vi "main functie.vi"(11 "input array   4":dbl[](array[numeric])) -> (2 "Array":i32[](array[numeric]), 3 "Numeric":i32)   [LabVIEW 2019]
uses:
  <vilib>/myRIO/Common/Instrument Driver Framework/Utilities/typedefs/Analog Scaling Constants.ctl
  <vilib>/myRIO/Common/Instrument Driver Framework/Utilities/typedefs/Analog Scaling Constants List.ctl
  <vilib>/myRIO/Common/Instrument Driver Framework/myRIO v1.0/AO/typedefs/AO Channels Enum.ctl
  <vilib>/myRIO/Common/Instrument Driver Framework/myRIO v1.0/AO/typedefs/AO Channels List.ctl
  <vilib>/myRIO/Common/Instrument Driver Framework/Utilities/typedefs/Generic FPGA Reference.ctl
  <vilib>/myRIO/Common/Instrument Driver Framework/Utilities/typedefs/myRIO v1.0 Reference.ctl
  <vilib>/myRIO/Common/Instrument Driver Framework/Utilities/typedefs/Hardware Version Enum.ctl
  <vilib>/myRIO/Common/Instrument Driver Framework/Utilities/typedefs/myRIO Generic Hardware Reference.ctl
  <vilib>/myRIO/Instrument Drivers/Onboard IO/AO/typedefs/AO Reference.ctl
  <vilib>/myRIO/Instrument Drivers/Onboard IO/AO/AO.lvlib
  <vilib>/myRIO/Instrument Drivers/Onboard IO/AO/vis/Write.vi
  <vilib>/userDefined/High Color/nirio_resource_hc.ctl
  <vilib>/myRIO/Common/Instrument Driver Framework/myRIO v1.0/AO/vis/myRIO v1.1 Open AO.vi
  <vilib>/myRIO/Instrument Drivers/Onboard IO/AO/vis/myRIO AO Open.xnode
  <vilib>/myRIO/Common/Instrument Driver Framework/Utilities/vis/Is FPGA Ref Available.vi
  <vilib>/myRIO/Express VI/Onboard IO/AO/AO Express VI.xnode
panel:
  in  "Numeric 4":dbl
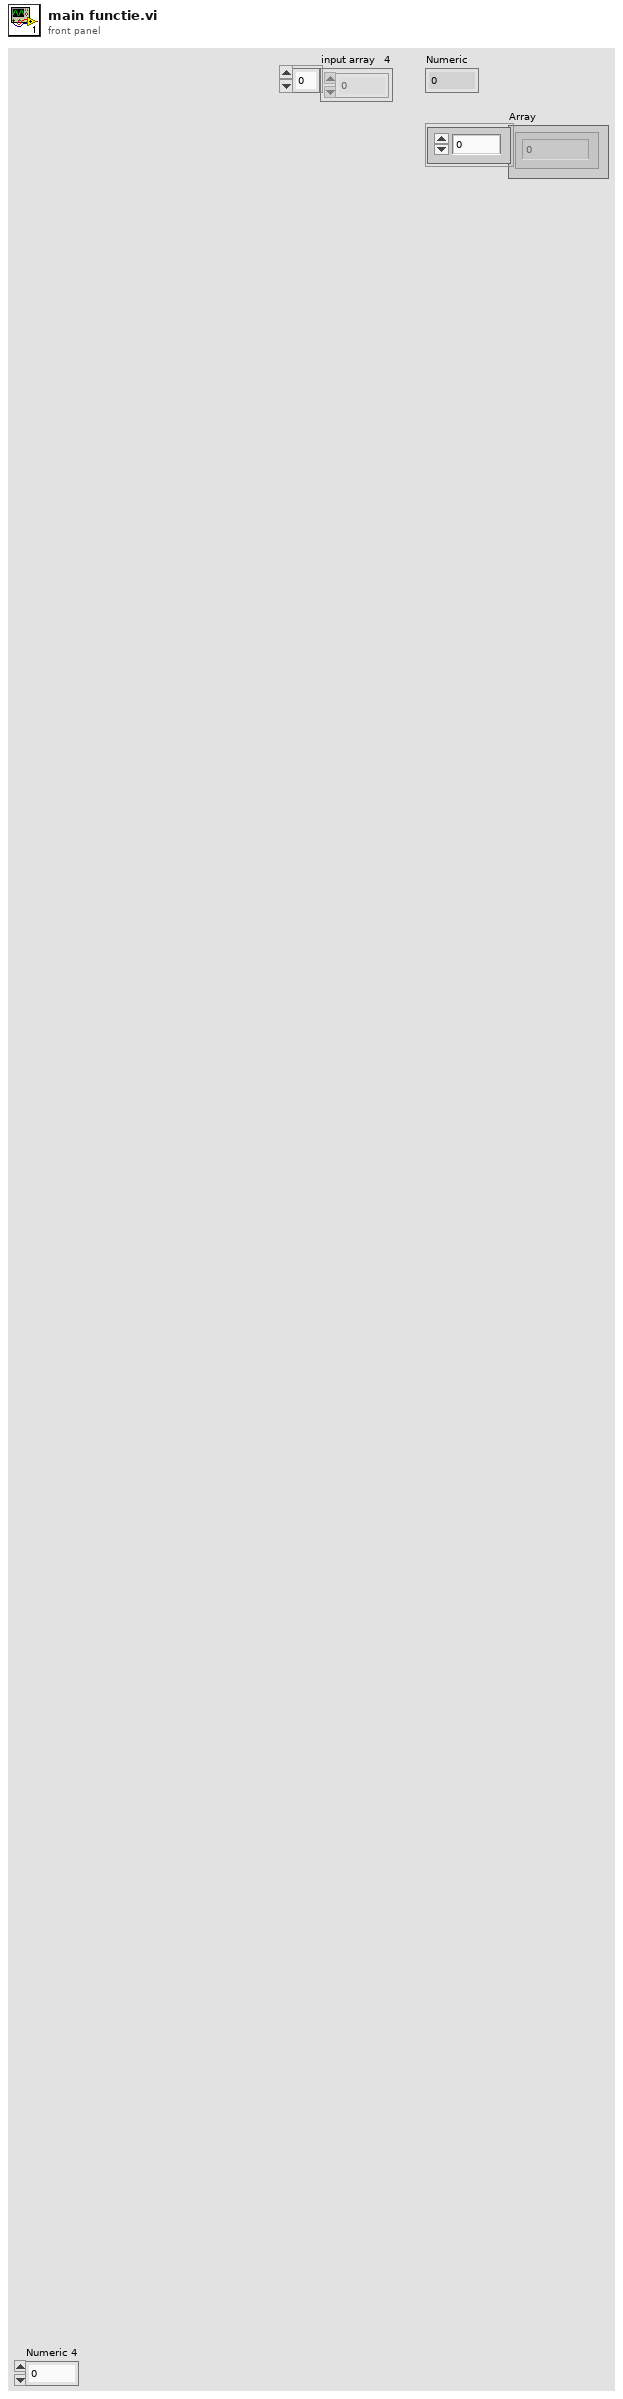
[diagram p1: front panel]
types:
  T1 = typedef "AO.lvlib/AO Reference.ctl" = cluster{"myRIO Reference":T2, "AO Channel List":T6, "AO Scaling Constant List":T8}
  T2 = typedef "myRIO Generic Hardware Reference.ctl" = cluster{"myRIO Model":T3, "myRIO Hardware Reference":T4}
  T3 = typedef "Hardware Version Enum.ctl" = enum16{"Unknown", "myRIO-1900", "myRIO-1950", "roboRIO", "NI ELVIS RIO CM", "ELVIS III"}
  T4 = typedef "myRIO v1.0 Reference.ctl" = cluster{"Generic FPGA Reference":T5, "Allow multiple opens":bool}
  T5 = typedef "Generic FPGA Reference.ctl" = refnum<k20>
  T6 = typedef "AO Channels List.ctl" = T7[]
  T7 = typedef "AO Channels Enum.ctl" = enum16{"Not Connected", "AudioOut/Left", "AudioOut/Right", "C/AO0", "C/AO1", "A/AO0", "A/AO1", "B/AO0", "B/AO1"}
  T8 = typedef "Analog Scaling Constants List.ctl" = T9[]
  T9 = typedef "Analog Scaling Constants.ctl" = cluster{"LSB Weight (Volts)":dbl, "Offset (Volts)":dbl, "Signed?":bool}
  T10 = typedef "nirio_resource_hc.ctl" = tag
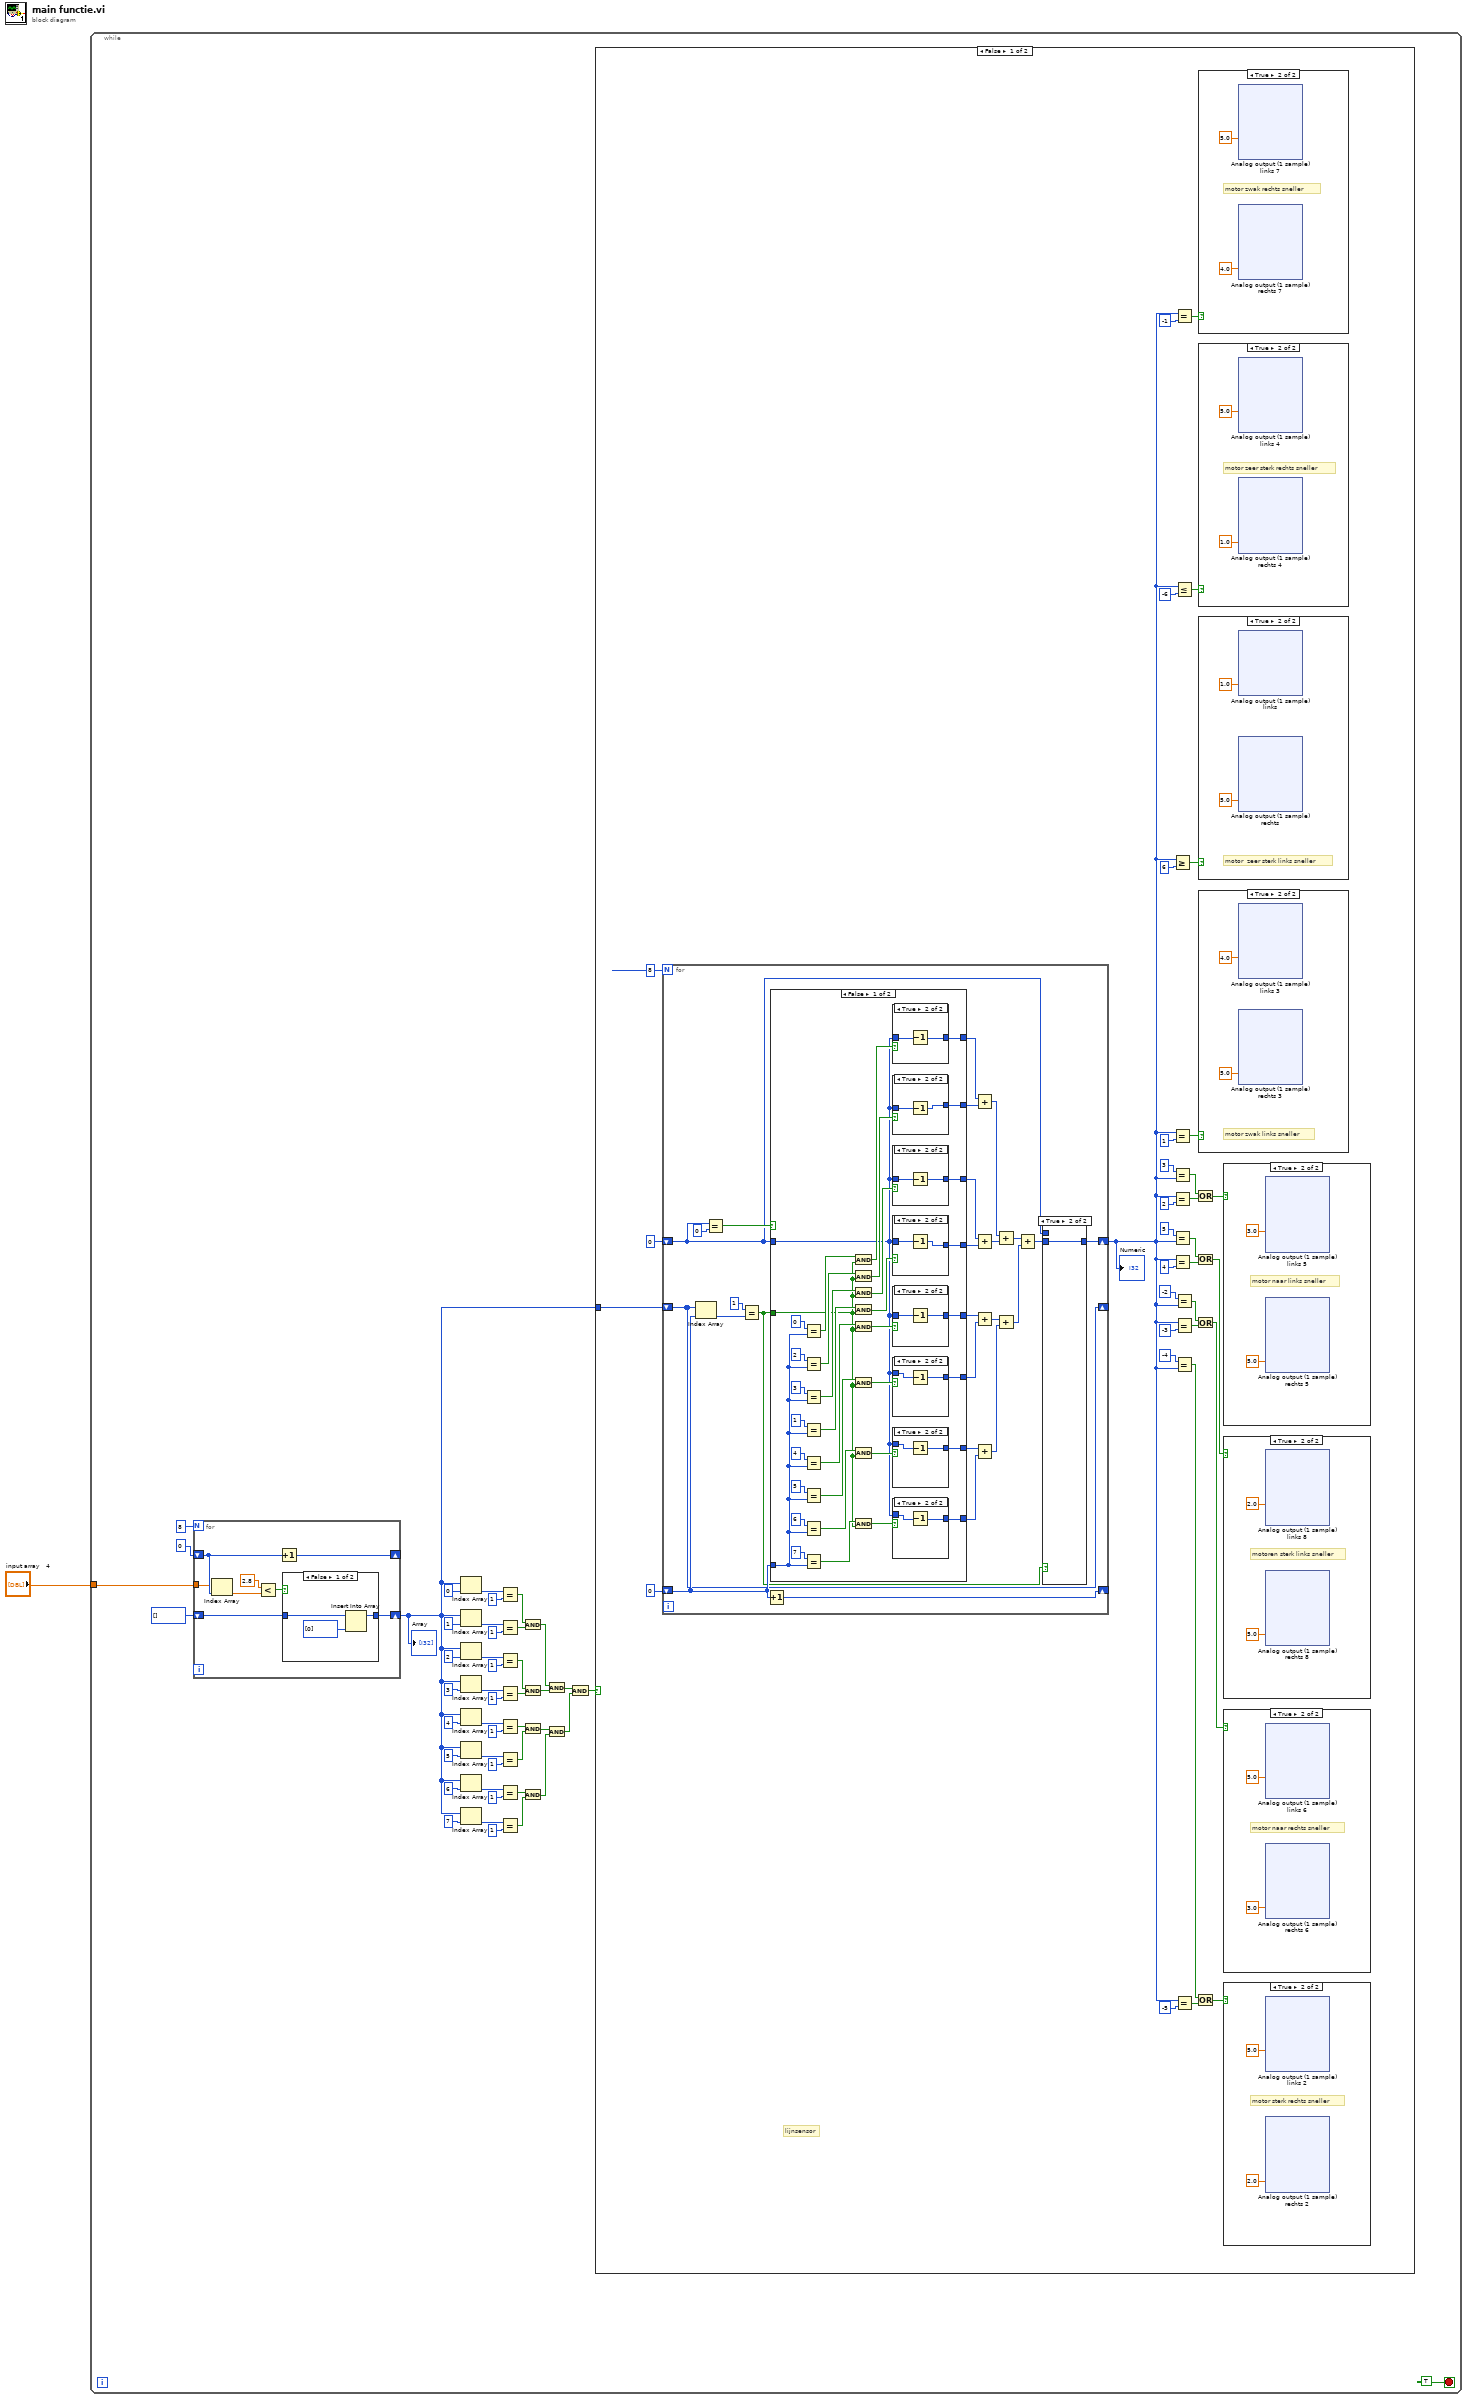
[diagram p0: block diagram]
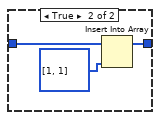
[diagram p2: hidden frame]
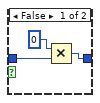
[diagram p12: hidden frame]
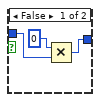
[diagram p13: hidden frame]
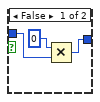
[diagram p14: hidden frame]
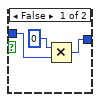
[diagram p15: hidden frame]
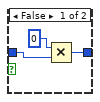
[diagram p16: hidden frame]
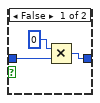
[diagram p17: hidden frame]
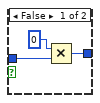
[diagram p18: hidden frame]
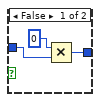
[diagram p19: hidden frame]
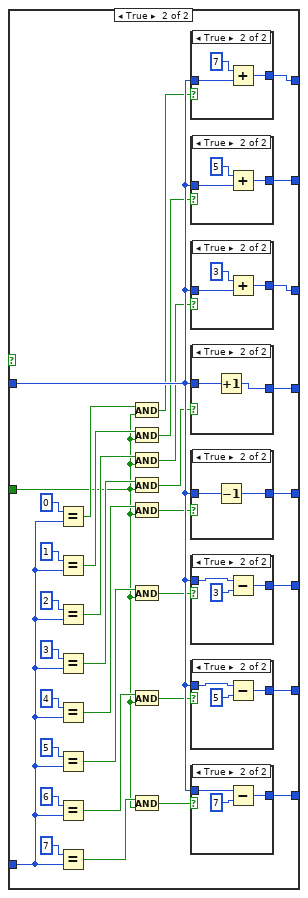
[diagram p20: hidden frame]
diagram:
  n1 = while {
    tunnel: "input array   4" -> [w46]
    stop <- TRUE stop-if-true
    n2 = for {
      N: 8 -> [_]
      shift-right: [w53] -> w45
      shift-left: i32[] [] -> [w54]
      shift-right: [w50] -> _
      shift-left: 0 -> [w49]
      tunnel: w46 -> [w47]
      n3 = Index Array(array=w47, index=w49) -> (element=w48:dbl)
      n4 = Less?(x=2.8, y=w48) -> (x < y?=w52:bool)
      n5 = Increment(x=w49) -> (x+1=w50:i32)
      n6 = case shown="False" w52 {
        tunnel: w54 -> [w56 w58]
        tunnel: [w57 w60] -> w53
        frame False {
          n7 = Insert Into Array(array=w56, new element=i32[] [0]) -> (w57:i32[])  [unwired: 1 in]
        }
        frame True {
          n8 = Insert Into Array(array=w58, new element=i32[] [1, 1]) -> (w60:i32[])  [unwired: 1 in]
        }
      }
    }
    "Array" <- w45
    n9 = Index Array(array=w45, index=0) -> (element=w24:i32)
    n10 = Index Array(array=w45, index=1) -> (element=w3:i32)
    n11 = Index Array(array=w45, index=2) -> (element=w9:i32)
    n12 = Index Array(array=w45, index=3) -> (element=w6:i32)
    n13 = Index Array(array=w45, index=4) -> (element=w12:i32)
    n14 = Index Array(array=w45, index=5) -> (element=w15:i32)
    n15 = Index Array(array=w45, index=6) -> (element=w18:i32)
    n16 = Index Array(array=w45, index=7) -> (element=w21:i32)
    n17 = Equal?(x=w24, y=1) -> (x = y?=w27:bool)
    n18 = Equal?(x=w3, y=1) -> (x = y?=w28:bool)
    n19 = Equal?(x=w9, y=1) -> (x = y?=w29:bool)
    n20 = Equal?(x=w6, y=1) -> (x = y?=w30:bool)
    n21 = Equal?(x=w12, y=1) -> (x = y?=w31:bool)
    n22 = Equal?(x=w15, y=1) -> (x = y?=w32:bool)
    n23 = Equal?(x=w18, y=1) -> (x = y?=w33:bool)
    n24 = Equal?(x=w21, y=1) -> (x = y?=w34:bool)
    n25 = And(x=w27, y=w28) -> (x .and. y?=w35:bool)
    n26 = And(x=w29, y=w30) -> (x .and. y?=w36:bool)
    n27 = And(x=w31, y=w32) -> (x .and. y?=w37:bool)
    n28 = And(x=w33, y=w34) -> (x .and. y?=w38:bool)
    n29 = And(x=w35, y=w36) -> (x .and. y?=w39:bool)
    n30 = And(x=w37, y=w38) -> (x .and. y?=w40:bool)
    n31 = And(x=w39, y=w40) -> (x .and. y?=w41:bool)
    n32 = case shown="False" w41 {
      tunnel: w45 -> [w62 _]
      frame False {
        # "lijnsensor"
        n33 = for {
          N: 8 -> [_]
          shift-right: [w712] -> _
          shift-left: 0 -> [w726]
          shift-right: [w704] -> w61
          shift-left: 0 -> [w705]
          shift-right: [w717] -> _
          shift-left: w62 -> [w717]
          n34 = Index Array(array=w717, index=w726) -> (element=w716:i32)
          n35 = Equal?(x=w705, y=0) -> (x = y?=w713:bool)
          n36 = Equal?(x=1, y=w716) -> (x = y?=w703:bool)
          n37 = Increment(x=w726) -> (x+1=w712:i32)
          n38 = case shown="False" w713 {
            tunnel: w726 -> [w736 w822]
            tunnel: [w730 w821] -> w725
            tunnel: [w737 w820] -> w724
            tunnel: [w738 w819] -> w723
            tunnel: [w739 w818] -> w722
            tunnel: w705 -> [w729 w817]
            tunnel: w703 -> [w735 w808]
            tunnel: [w733 w807] -> w711
            tunnel: [w734 w806] -> w710
            tunnel: [w731 w805] -> w708
            tunnel: [w732 w804] -> w707
            frame False {
              n39 = Equal?(x=0, y=w736) -> (x = y?=w756:bool)
              n40 = Equal?(x=2, y=w736) -> (x = y?=w762:bool)
              n41 = Equal?(x=3, y=w736) -> (x = y?=w763:bool)
              n42 = Equal?(x=1, y=w736) -> (x = y?=w748:bool)
              n43 = Equal?(x=4, y=w736) -> (x = y?=w760:bool)
              n44 = Equal?(x=5, y=w736) -> (x = y?=w761:bool)
              n45 = Equal?(x=6, y=w736) -> (x = y?=w759:bool)
              n46 = Equal?(x=7, y=w736) -> (x = y?=w758:bool)
              n47 = And(x=w756, y=w735) -> (x .and. y?=w740:bool)
              n48 = And(x=w762, y=w735) -> (x .and. y?=w742:bool)
              n49 = And(x=w763, y=w735) -> (x .and. y?=w743:bool)
              n50 = And(x=w748, y=w735) -> (x .and. y?=w741:bool)
              n51 = And(x=w760, y=w735) -> (x .and. y?=w744:bool)
              n52 = And(x=w761, y=w735) -> (x .and. y?=w745:bool)
              n53 = And(x=w759, y=w735) -> (x .and. y?=w746:bool)
              n54 = And(x=w758, y=w735) -> (x .and. y?=w747:bool)
              n55 = case shown="True" w740 {
                tunnel: [w765 w768] -> w734
                tunnel: w729 -> [w764 w767]
                frame False {
                  n56 = Multiply(x=0, y=w764) -> (x*y=w765:i32)
                }
                frame True {
                  n57 = Decrement(x=w767) -> (x-1=w768:i32)
                }
              }
              n58 = case shown="True" w742 {
                tunnel: [w796 w797] -> w733
                tunnel: w729 -> [w795 w798]
                frame False {
                  n59 = Multiply(x=0, y=w795) -> (x*y=w796:i32)
                }
                frame True {
                  n60 = Decrement(x=w798) -> (x-1=w797:i32)
                }
              }
              n61 = case shown="True" w743 {
                tunnel: [w790 w793] -> w732
                tunnel: w729 -> [w789 w792]
                frame False {
                  n62 = Multiply(x=0, y=w789) -> (x*y=w790:i32)
                }
                frame True {
                  n63 = Decrement(x=w792) -> (x-1=w793:i32)
                }
              }
              n64 = case shown="True" w741 {
                tunnel: [w800 w803] -> w731
                tunnel: w729 -> [w799 w802]
                frame False {
                  n65 = Multiply(x=0, y=w799) -> (x*y=w800:i32)
                }
                frame True {
                  n66 = Decrement(x=w802) -> (x-1=w803:i32)
                }
              }
              n67 = case shown="True" w744 {
                tunnel: [w785 w788] -> w730
                tunnel: w729 -> [w784 w787]
                frame False {
                  n68 = Multiply(x=0, y=w784) -> (x*y=w785:i32)
                }
                frame True {
                  n69 = Decrement(x=w787) -> (x-1=w788:i32)
                }
              }
              n70 = case shown="True" w745 {
                tunnel: [w775 w778] -> w737
                tunnel: w729 -> [w774 w777]
                frame False {
                  n71 = Multiply(x=0, y=w774) -> (x*y=w775:i32)
                }
                frame True {
                  n72 = Decrement(x=w777) -> (x-1=w778:i32)
                }
              }
              n73 = case shown="True" w746 {
                tunnel: [w780 w783] -> w738
                tunnel: w729 -> [w779 w782]
                frame False {
                  n74 = Multiply(x=0, y=w779) -> (x*y=w780:i32)
                }
                frame True {
                  n75 = Decrement(x=w782) -> (x-1=w783:i32)
                }
              }
              n76 = case shown="True" w747 {
                tunnel: [w769 w773] -> w739
                tunnel: w729 -> [w770 w772]
                frame False {
                  n77 = Multiply(x=0, y=w770) -> (x*y=w769:i32)
                }
                frame True {
                  n78 = Decrement(x=w772) -> (x-1=w773:i32)
                }
              }
            }
            frame True {
              n79 = Equal?(x=0, y=w822) -> (x = y?=w831:bool)
              n80 = Equal?(x=1, y=w822) -> (x = y?=w823:bool)
              n81 = Equal?(x=2, y=w822) -> (x = y?=w837:bool)
              n82 = Equal?(x=3, y=w822) -> (x = y?=w838:bool)
              n83 = Equal?(x=4, y=w822) -> (x = y?=w835:bool)
              n84 = Equal?(x=5, y=w822) -> (x = y?=w836:bool)
              n85 = Equal?(x=6, y=w822) -> (x = y?=w834:bool)
              n86 = Equal?(x=7, y=w822) -> (x = y?=w833:bool)
              n87 = And(x=w831, y=w808) -> (x .and. y?=w809:bool)
              n88 = And(x=w823, y=w808) -> (x .and. y?=w810:bool)
              n89 = And(x=w837, y=w808) -> (x .and. y?=w811:bool)
              n90 = And(x=w838, y=w808) -> (x .and. y?=w812:bool)
              n91 = And(x=w835, y=w808) -> (x .and. y?=w813:bool)
              n92 = And(x=w836, y=w808) -> (x .and. y?=w814:bool)
              n93 = And(x=w834, y=w808) -> (x .and. y?=w815:bool)
              n94 = And(x=w833, y=w808) -> (x .and. y?=w816:bool)
              n95 = case shown="True" w809 {
                tunnel: w817 -> [w839 w843]
                tunnel: [w840 w842] -> w806
                frame False {
                  n96 = Multiply(x=0, y=w839) -> (x*y=w840:i32)
                }
                frame True {
                  n97 = Add(x=7, y=w843) -> (x+y=w842:i32)
                }
              }
              n98 = case shown="True" w810 {
                tunnel: w817 -> [w879 w882]
                tunnel: [w880 w883] -> w807
                frame False {
                  n99 = Multiply(x=0, y=w879) -> (x*y=w880:i32)
                }
                frame True {
                  n100 = Add(x=5, y=w882) -> (x+y=w883:i32)
                }
              }
              n101 = case shown="True" w811 {
                tunnel: w817 -> [w873 w877]
                tunnel: [w874 w876] -> w804
                frame False {
                  n102 = Multiply(x=0, y=w873) -> (x*y=w874:i32)
                }
                frame True {
                  n103 = Add(x=3, y=w877) -> (x+y=w876:i32)
                }
              }
              n104 = case shown="True" w812 {
                tunnel: w817 -> [w869 w872]
                tunnel: [w868 w871] -> w805
                frame False {
                  n105 = Multiply(x=0, y=w869) -> (x*y=w868:i32)
                }
                frame True {
                  n106 = Increment(x=w872) -> (x+1=w871:i32)
                }
              }
              n107 = case shown="True" w813 {
                tunnel: w817 -> [w863 w867]
                tunnel: [w864 w866] -> w821
                frame False {
                  n108 = Multiply(x=0, y=w863) -> (x*y=w864:i32)
                }
                frame True {
                  n109 = Decrement(x=w867) -> (x-1=w866:i32)
                }
              }
              n110 = case shown="True" w814 {
                tunnel: w817 -> [w852 w854]
                tunnel: [w851 w856] -> w820
                frame False {
                  n111 = Multiply(x=0, y=w852) -> (x*y=w851:i32)
                }
                frame True {
                  n112 = Subtract(x=w854, y=3) -> (x-y=w856:i32)
                }
              }
              n113 = case shown="True" w815 {
                tunnel: w817 -> [w858 w860]
                tunnel: [w857 w861] -> w819
                frame False {
                  n114 = Multiply(x=0, y=w858) -> (x*y=w857:i32)
                }
                frame True {
                  n115 = Subtract(x=w860, y=5) -> (x-y=w861:i32)
                }
              }
              n116 = case shown="True" w816 {
                tunnel: w817 -> [w845 w848]
                tunnel: [w846 w849] -> w818
                frame False {
                  n117 = Multiply(x=0, y=w845) -> (x*y=w846:i32)
                }
                frame True {
                  n118 = Subtract(x=w848, y=7) -> (x-y=w849:i32)
                }
              }
            }
          }
          n119 = Add(x=w710, y=w711) -> (x+y=w709:i32)
          n120 = Add(x=w707, y=w708) -> (x+y=w706:i32)
          n121 = Add(x=w725, y=w724) -> (x+y=w720:i32)
          n122 = Add(x=w723, y=w722) -> (x+y=w721:i32)
          n123 = Add(x=w709, y=w706) -> (x+y=w719:i32)
          n124 = Add(x=w720, y=w721) -> (x+y=w718:i32)
          n125 = Add(x=w719, y=w718) -> (x+y=w702:i32)
          n126 = case shown="True" w703 {
            tunnel: w705 -> [w727 _]
            tunnel: [w727 w728] -> w704
            tunnel: w702 -> [_ w728]
            frame False {
            }
            frame True {
            }
          }
        }
        "Numeric" <- w61
        n127 = Greater Or Equal?(x=w61, y=6) -> (x >= y?=w88:bool)
        n128 = Equal?(x=w61, y=1) -> (x = y?=w89:bool)
        n129 = Equal?(x=3, y=w61) -> (x = y?=w79:bool)
        n130 = Equal?(x=w61, y=2) -> (x = y?=w80:bool)
        n131 = Equal?(x=5, y=w61) -> (x = y?=w83:bool)
        n132 = Equal?(x=w61, y=4) -> (x = y?=w84:bool)
        n133 = Equal?(x=w61, y=-1) -> (x = y?=w67:bool)
        n134 = Less Or Equal?(x=w61, y=-6) -> (x <= y?=w65:bool)
        n135 = Equal?(x=-2, y=w61) -> (x = y?=w73:bool)
        n136 = Equal?(x=w61, y=-3) -> (x = y?=w74:bool)
        n137 = Equal?(x=-4, y=w61) -> (x = y?=w69:bool)
        n138 = Equal?(x=w61, y=-5) -> (x = y?=w70:bool)
        n139 = Or(x=w79, y=w80) -> (x .or. y?=w77:bool)
        n140 = Or(x=w83, y=w84) -> (x .or. y?=w85:bool)
        n141 = Or(x=w73, y=w74) -> (x .or. y?=w66:bool)
        n142 = Or(x=w69, y=w70) -> (x .or. y?=w63:bool)
        n143 = case shown="True" w67 {
          frame False {
          }
          frame True {
            # "motor zwak rechts sneller"
            n144 = xnode "Analog output (1 sample) links 7"("A/AO0 (Pin 2)"=5.0) -> ()  [unwired: 1 in, 1 out]
            n145 = xnode "Analog output (1 sample) rechts 7"("A/AO0 (Pin 2)"=4.0) -> ()  [unwired: 1 in, 1 out]
          }
        }
        n146 = case shown="True" w65 {
          frame False {
          }
          frame True {
            # "motor zeer sterk rechts sneller"
            n147 = xnode "Analog output (1 sample) links 4"("A/AO0 (Pin 2)"=5.0) -> ()  [unwired: 1 in, 1 out]
            n148 = xnode "Analog output (1 sample) rechts 4"("A/AO0 (Pin 2)"=1.0) -> ()  [unwired: 1 in, 1 out]
          }
        }
        n149 = case shown="True" w88 {
          frame False {
          }
          frame True {
            # "motor  zeer sterk links sneller"
            n150 = xnode "Analog output (1 sample) links"("A/AO0 (Pin 2)"=1.0) -> ()  [unwired: 1 in, 1 out]
            n151 = xnode "Analog output (1 sample) rechts"("A/AO0 (Pin 2)"=5.0) -> ()  [unwired: 1 in, 1 out]
          }
        }
        n152 = case shown="True" w89 {
          frame False {
          }
          frame True {
            # "motor zwak links sneller"
            n153 = xnode "Analog output (1 sample) links 3"("A/AO0 (Pin 2)"=4.0) -> ()  [unwired: 1 in, 1 out]
            n154 = xnode "Analog output (1 sample) rechts 3"("A/AO0 (Pin 2)"=5.0) -> ()  [unwired: 1 in, 1 out]
          }
        }
        n155 = case shown="True" w77 {
          frame False {
          }
          frame True {
            # "motor naar links sneller"
            n156 = xnode "Analog output (1 sample) links 5"("A/AO0 (Pin 2)"=3.0) -> ()  [unwired: 1 in, 1 out]
            n157 = xnode "Analog output (1 sample) rechts 5"("A/AO0 (Pin 2)"=5.0) -> ()  [unwired: 1 in, 1 out]
          }
        }
        n158 = case shown="True" w85 {
          frame False {
          }
          frame True {
            # "motoren sterk links sneller"
            n159 = xnode "Analog output (1 sample) links 8"("A/AO0 (Pin 2)"=2.0) -> ()  [unwired: 1 in, 1 out]
            n160 = xnode "Analog output (1 sample) rechts 8"("A/AO0 (Pin 2)"=5.0) -> ()  [unwired: 1 in, 1 out]
          }
        }
        n161 = case shown="True" w66 {
          frame False {
          }
          frame True {
            # "motor naar rechts sneller"
            n162 = xnode "Analog output (1 sample) links 6"("A/AO0 (Pin 2)"=5.0) -> ()  [unwired: 1 in, 1 out]
            n163 = xnode "Analog output (1 sample) rechts 6"("A/AO0 (Pin 2)"=3.0) -> ()  [unwired: 1 in, 1 out]
          }
        }
        n164 = case shown="True" w63 {
          frame False {
          }
          frame True {
            # "motor sterk rechts sneller"
            n165 = xnode "Analog output (1 sample) links 2"("A/AO0 (Pin 2)"=5.0) -> ()  [unwired: 1 in, 1 out]
            n166 = xnode "Analog output (1 sample) rechts 2"("A/AO0 (Pin 2)"=2.0) -> ()  [unwired: 1 in, 1 out]
          }
        }
      }
      frame True {
        n167 = feedback #1() -> (w885:i32)  [unwired: 1 in]
        n168 = Equal?(x=w885, y=0) -> (x = y?=w887:bool)
        n169 = case shown="False" w887 {
          tunnel: [1 1] -> w886
          frame False {
            n170 = In Range and Coerce(upper limit=660, x="Numeric 4", lower limit=460) -> (In Range?=w889:bool)  [unwired: 1 out]
            n171 = case shown="True" w889 {
              frame False {
              }
              frame True {
                n172 = case shown="False" TRUE {
                  selector: TRUE -> [w896 _]
                  tunnel: [w896 _] -> _
                  frame False {
                    n173 = case shown="False" TRUE {
                      frame False {
                        # "links bocht"
                        n174 = xnode "Analog output (1 sample) 7"("A/AO0 (Pin 2)"=1.0) -> ()  [unwired: 1 in, 1 out]
                        n175 = xnode "Analog output (1 sample) 8"("A/AO0 (Pin 2)"=5.0) -> ()  [unwired: 1 in, 1 out]
                      }
                      frame True {
                        # "rechts bocht"
                        n176 = xnode "Analog output (1 sample) 4"("A/AO0 (Pin 2)"=5.0) -> ()  [unwired: 1 in, 1 out]
                        n177 = xnode "Analog output (1 sample) 3"("A/AO0 (Pin 2)"=1.0) -> ()  [unwired: 1 in, 1 out]
                      }
                    }
                  }
                  frame True {
                    # "rechtdoor"
                    n178 = xnode "Analog output (1 sample) 5"("A/AO0 (Pin 2)"=5.0) -> ()  [unwired: 1 in, 1 out]
                    n179 = xnode "Analog output (1 sample) 6"("A/AO0 (Pin 2)"=5.0) -> ()  [unwired: 1 in, 1 out]
                  }
                }
              }
            }
          }
          frame True {
            w1126 = 0.0
            # "motor  stilleggen"
            n180 = xnode "Analog output (1 sample)"("A/AO0 (Pin 2)"=w1126) -> ()  [unwired: 1 in, 1 out]
            n181 = xnode "Analog output (1 sample) 2"("A/AO0 (Pin 2)"=w1126) -> ()  [unwired: 1 in, 1 out]
          }
        }
        n182 = feedback-in #1(w886) -> ()
      }
    }
  }
